vi "Apply.vi"(8 "error in (no error)":errorcluster, 9 "Fs (Hz)":dbl, 10 "Array in":dbl[](array[numeric]), 11 "AM in":refnum<class "AM.lvclass">) -> (0 "error out":errorcluster, 2 "Array out":dbl[](array[numeric]), 3 "AM out":refnum<class "AM.lvclass">)   [LabVIEW 2015, in "AM.lvclass"]
uses:
  AM.lvclass
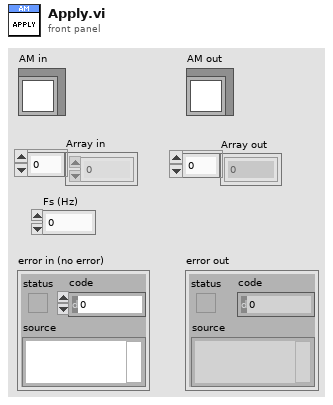
[diagram p1: front panel]
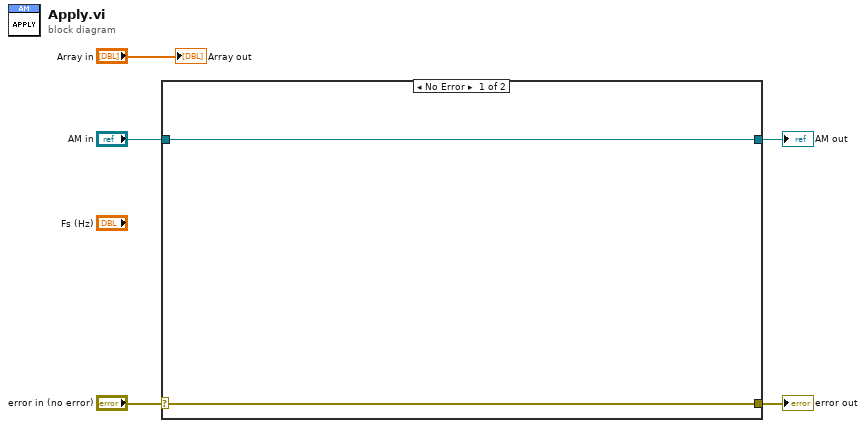
[diagram p0: block diagram]
diagram:
  n1 = case shown="No Error" "error in (no error)" {
    selector: "error in (no error)" -> [w6 w9]
    tunnel: [w6 w9] -> w4
    tunnel: [w7 w8] -> w2
    tunnel: "AM in" -> [w7 w8]
    frame No Error {
    }
    frame Error {
    }
  }
  "error out" <- w4
  "AM out" <- w2
  "Array out" <- "Array in"
